vi "Request and Wait for Reply Timeout--error.vi"(11 "Error Message":string) -> (0 "error out":errorcluster)   [LabVIEW 2020, in "UI.lvlib"]
doc: "Generate an error for the situation where the Request and Wait for Reply times out.\n_____\nBased on DQMH Dev Tools: Project Template 7.1.1.1528."
uses:
  UI.lvlib
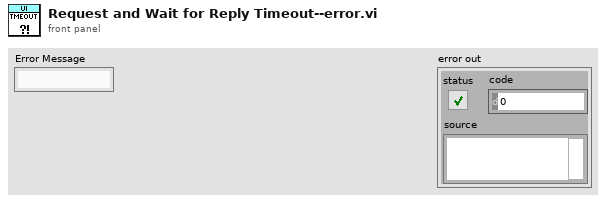
[diagram p1: front panel]
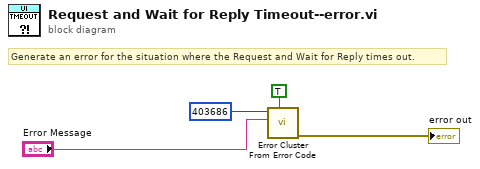
[diagram p0: block diagram]
diagram:
  # "Generate an error for the situation where the Request and Wait for Reply times out."
  n1 = call <vilib>:"Error Cluster From Error Code.vi"("show call chain? (False)"=TRUE, "error message (\"\")"="Error Message", "error code (0)"=403686) -> ("error out"=→"error out":errorcluster)  [unwired: 6 in]
